vi "Report Event.vi"(7 "Level (Info)":T1=enum."Info", 8 "error in (no error)":errorcluster, 9 "Message":string, 10 "Context":string, 11 "Event API in":refnum<class "EventAPI.lvclass">) -> (0 "error out":errorcluster, 3 "Event API out":refnum<class "EventAPI.lvclass">)   [LabVIEW 2020, in "Volatus.lvlib" / "EventAPI.lvclass"]
uses:
  EventAPI.lvclass
  Event Level.ctl
  EventAPI.lvclass/EventAPI.ctl
  Event.ctl
  EventHandler Messages/Handle Event Msg/Handle Event Msg.lvclass/Handle Event Msg.ctl
  <vilib>/ActorFramework/Message Enqueuer/Message Enqueuer.lvclass/Message Enqueuer.ctl
  <vilib>/ActorFramework/Message Enqueuer/Enqueue.vi
  EventHandler Messages/Handle Event Msg/Handle Event Msg.lvclass
  C:/Program Files (x86)/National Instruments/LabVIEW 2020/vi.lib/ActorFramework/Message/Message.lvclass
  <vilib>/ActorFramework/Message Priority Queue/Priority Enqueue.vi
  Volatus.lvlib
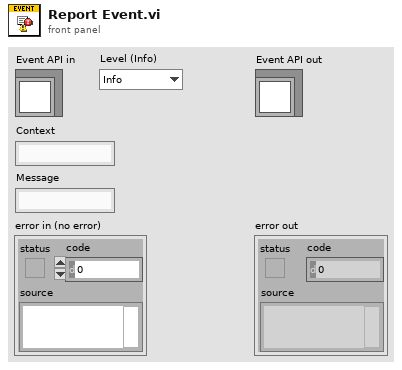
[diagram p1: front panel]
types:
  T1 = typedef "Volatus.lvlib/Event Level.ctl" = enum16{"Debug", "Info", "Warning", "Error"}
  T2 = typedef "Volatus.lvlib/Event.ctl" = cluster{"Level":T1, "Context":string, "Message":string, "Error":errorcluster, "Time Stamp":timestamp}
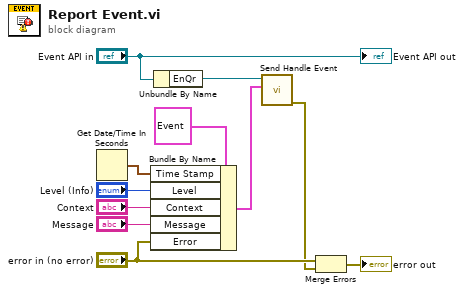
[diagram p0: block diagram]
diagram:
  n1 = Get Date/Time In Seconds() -> (seconds since 1Jan1904=w1:timestamp)
  n2 = Bundle By Name(cluster=T2 {"Level"=enum."Info", "Context"="", "Message"="", "Error"={"status"=FALSE, "code"=0, "source"=""}, "Time Stamp"=timestamp(0 s since 1904-01-01)} ("Event"), "Time Stamp"=w1, "Level"="Level (Info)", "Context"="Context", "Message"="Message", "Error"="error in (no error)") -> (w4:T2)
  n3 = Unbundle By Name("Event API in") -> ("EnQr"=w5:refnum<class "Message Enqueuer.lvclass">)
  n4 = call "Send Handle Event.vi"("Event"=w4, "Message Enqueuer"=w5) -> ("error out"=w2:errorcluster)  [unwired: 8 in, 1 out]
  n5 = Merge Errors("error in (no error)", w2) -> (→"error out":errorcluster)
  "Event API out" <- "Event API in"
